vi "Write to Config.vi"(8 "error in (no error)":errorcluster, 9 "Additional Data":string, 10 "Command":T1, 11 "Plugin Name":string) -> (0 "error out":errorcluster)   [LabVIEW 2021, in "CIFLogs.lvlib"]
uses:
  CIFLogs.lvlib
  Typedef/Plugin State Commands.ctl
  <vilib>/CIF Foundation/CIF Utilities/Time/System Time/LabVIEW Time to TAI Time.vi
  Typedef/Message Type.ctl
  <vilib>/CIF Foundation/CIF Utilities/Time/Time_CIF_U.lvlib
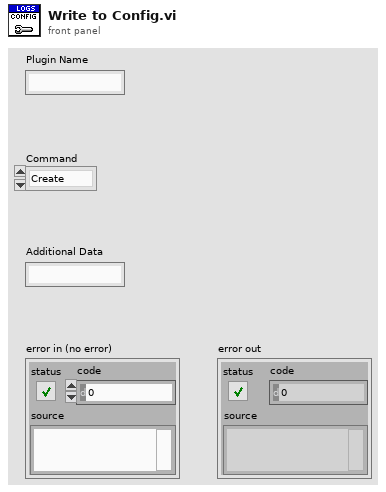
[diagram p1: front panel]
types:
  T1 = typedef "CIFLogs.lvlib/Plugin State Commands.ctl" = enum16{"Create", "Configure", "Run", "Pause", "Destroy", "Connect", "Force"}
  T2 = typedef "CIFLogs.lvlib/Message Type.ctl" = enum16{"Error", "Information", "Print Terminal", "Configuration"}
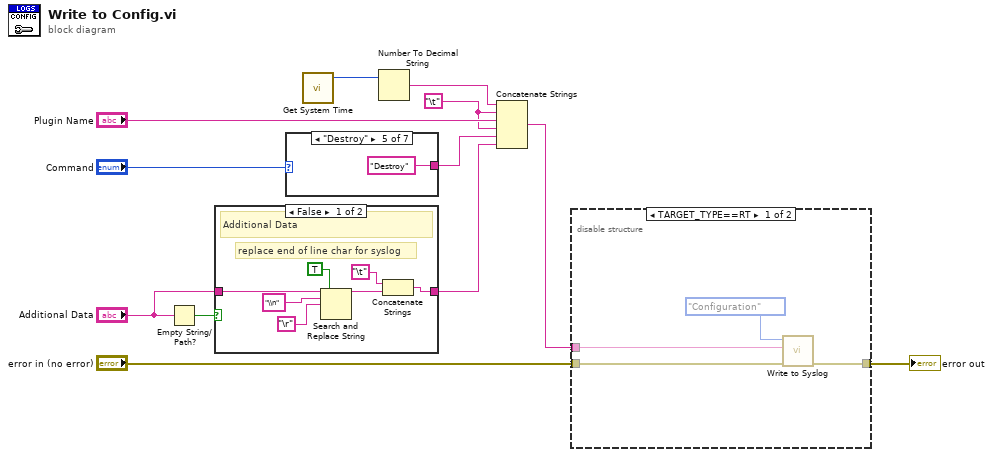
[diagram p0: block diagram]
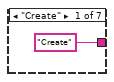
[diagram p3: hidden frame]
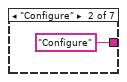
[diagram p4: hidden frame]
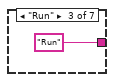
[diagram p5: hidden frame]
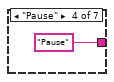
[diagram p6: hidden frame]
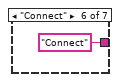
[diagram p7: hidden frame]
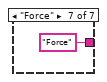
[diagram p8: hidden frame]
diagram:
  w3 = "\t"
  n1 = Empty String/Path?(string/path="Additional Data") -> (empty?=w5:bool)
  n2 = case shown="False" w5 {
    tunnel: "Additional Data" -> [w16 w20]
    tunnel: [w13 w20] -> w4
    frame False {
      # "replace end of line char for syslog"
      # "Additional Data"
      n3 = Search and Replace String(replace all?=TRUE ("replace all? (F)"), input string=w16, search string="\\n", replace string="\r") -> (result string=w15:string)  [unwired: 4 in, 3 out]
      n4 = Concatenate Strings("\t", w15) -> (w13:string)
    }
    frame True {
    }
  }
  n5 = case shown="\"Destroy\"" "Command" {
    tunnel: ["Create" "Configure" "Run" "Pause" "Destroy" "Connect" "Force"] -> w7
    frame "Create" {
    }
    frame "Configure" {
    }
    frame "Run" {
    }
    frame "Pause" {
    }
    frame "Destroy" {
    }
    frame "Connect" {
    }
    frame "Force" {
    }
  }
  n6 = call <vilib>:"Get System Time.vi"() -> ("Time (ns)"=w1:i64)  [unwired: 5 in]
  n7 = Number To Decimal String(number=w1) -> (decimal integer string=w2:string)  [unwired: 1 in]
  n8 = Concatenate Strings(w2, w3, "Plugin Name", w3, w7, w4) -> (w9:string)
  n9 = disable-structure shown="TARGET_TYPE==RT" {
    disable-tunnel: "error in (no error)" -> [w31 _]
    disable-tunnel: [w30 _] -> w11
    disable-tunnel: w9 -> [w28 _]
    frame condition #0 {
      n10 = call "Write to Syslog.vi"("error in (no error)"=w31, "message"=w28, "CIF Message Type"=Message_Type."Configuration") -> ("error out"=w30:errorcluster)  [unwired: 8 in]
    }
    frame condition #1 (active) {
    }
  }
  "error out" <- w11
